vi "2.vi"() -> ()   [LabVIEW 2020]
panel:
  in  "stop":bool
  in  "Value":dbl
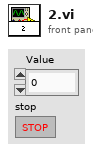
[diagram p1: front panel]
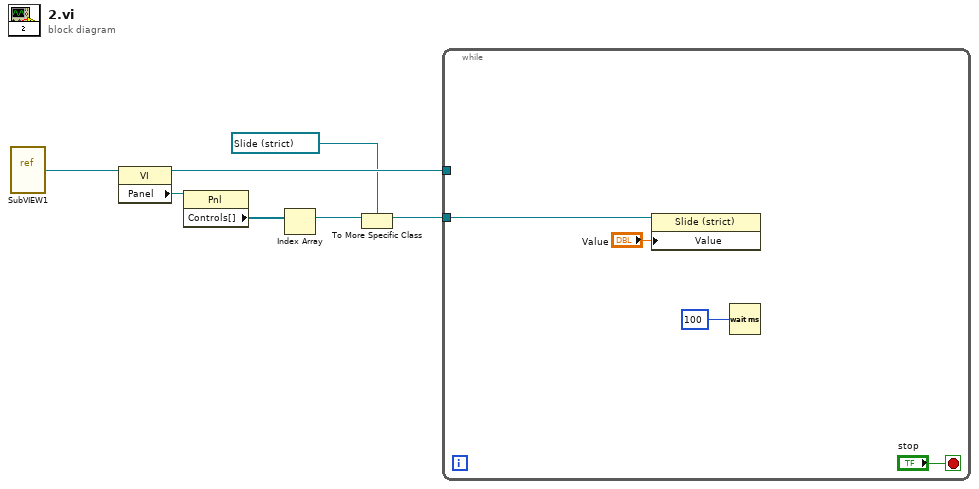
[diagram p0: block diagram]
diagram:
  n1 = vi-ref "SubVIEW1.vi"() -> (w7:refnum<vi>)
  n2 = property class="VI"(reference=w7) -> (reference out=w6:refnum<vi>, "Panel"=w5:refnum<vi>)  [unwired: 1 in, 1 out]
  n3 = property class="Pnl"(reference=w5) -> ("Controls[]"=w4:refnum<vi>[])  [unwired: 1 in, 2 out]
  n4 = Index Array(array=w4) -> (element=w3:refnum<vi>)  [unwired: 1 in]
  n5 = To More Specific Class(target class=refnum<vi> refnum ("高温泵压力#2"), reference=w3) -> (specific class reference=w2:refnum<vi>)  [unwired: 1 in, 1 out]
  n6 = while {
    tunnel: w6 -> [_]
    tunnel: w2 -> [w11]
    stop <- "stop" stop-if-true
    n7 = property class="Slide (strict)"(reference=w11, "Value"="Value") -> ()  [unwired: 1 in, 2 out]
    n8 = Wait (ms)(milliseconds to wait=u32 100 ("millisecond timer value")) -> ()  [unwired: 1 out]
  }
